vi "ep_Averaging Blocks.vi"(7 "reset":bool, 8 "error in (no error)":errorcluster, 11 "spectra parameters":T1) -> (0 "error out":errorcluster, 3 "averaging blocks":i32)   [LabVIEW 2014, in "NI_EP_Motor Monitoring.lvlib"]
uses:
  <vilib>/addons/Electrical Power/Motor Monitoring/NI_EP_Motor Monitoring.lvlib
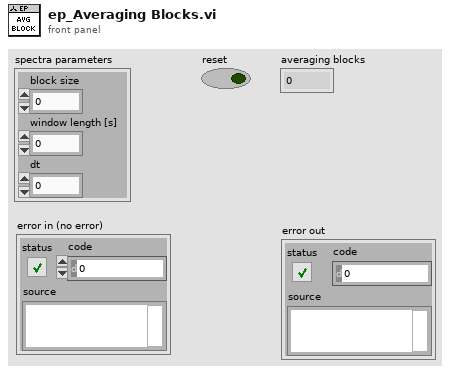
[diagram p1: front panel]
types:
  T1 = cluster{"block size":i32, "window length [s]":dbl, "dt":dbl}
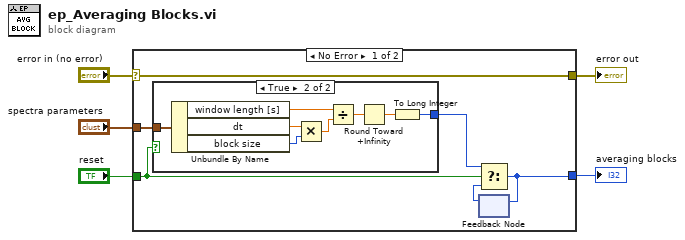
[diagram p0: block diagram]
diagram:
  n1 = case shown="No Error" "error in (no error)" {
    selector: "error in (no error)" -> [w11 w20]
    tunnel: [w11 w20] -> w4
    tunnel: [w7 _] -> w3
    tunnel: "reset" -> [w9 _]
    tunnel: "spectra parameters" -> [w6 _]
    frame No Error {
      n2 = case shown="True" w9 {
        tunnel: [_ w16] -> w8
        tunnel: w6 -> [_ w15]
        frame False {
        }
        frame True {
          n3 = Unbundle By Name(w15) -> ("window length [s]"=w14:dbl, "dt"=w13:dbl, "block size"=w12:i32)
          n4 = Multiply(x=w13, y=w12) -> (x*y=w19:dbl)
          n5 = Divide(x=w14, y=w19) -> (x/y=w18:dbl)
          n6 = Round Toward +Infinity(x=w18) -> (ceil(x): smallest int >= x=w17:dbl)
          n7 = To Long Integer(number=w17) -> (32bit integer=w16:i32)
        }
      }
      n8 = feedback #1() -> (w10:i32)  [unwired: 1 in]
      n9 = Select(t=w8, s=w9, f=w10) -> (s? t:f=w7:i32)
      n10 = feedback-in #1(w7) -> ()
    }
    frame Error {
    }
  }
  "error out" <- w4
  "averaging blocks" <- w3
